vi "USB Config low.vi"(0 "Port":refnum<visa-resource-name>, 1 "Tx msg cluster":T1={"dest"=1, "A/D/C/I"="A", "R/W"="R", "chan"=1, "val (float)"=0.0}, 2 "Error in":errorcluster) -> (3 "Port out":refnum<visa-resource-name>, 4 "Value returned":sgl, 6 "Error out":errorcluster)   [LabVIEW 2018]
uses:
  ctls/muCTA_USB Tx msg cluster.ctl
panel:
  out "Bytes returned":u32
  out "Read buffer (hex)":string
  out "Write buffer (hex)":string
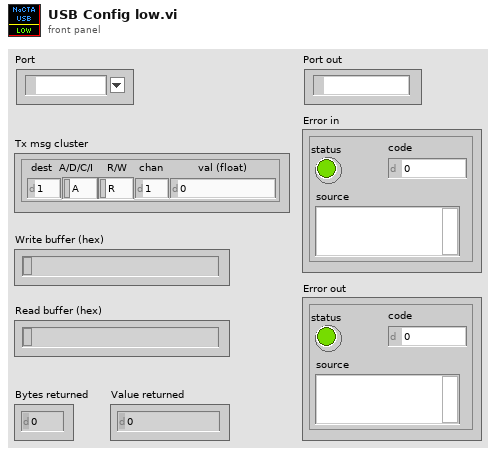
[diagram p1: front panel]
types:
  T1 = typedef "muCTA_USB Tx msg cluster.ctl" = cluster{"dest":u8, "A/D/C/I":string, "R/W":string, "chan":u8, "val (float)":sgl}
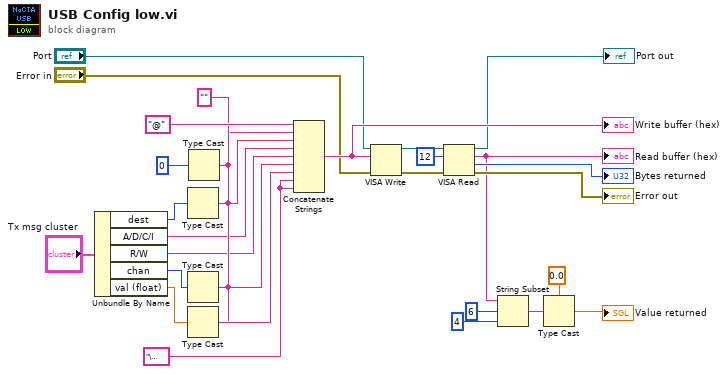
[diagram p0: block diagram]
diagram:
  w24 = "\u0000"
  w18 = ""
  n1 = Unbundle By Name("Tx msg cluster") -> ("dest"=w15:u8, "A/D/C/I"=w14:string, "R/W"=w13:string, "chan"=w12:u8, "val (float)"=w11:sgl)
  n2 = Type Cast(type=w18, x=w15) -> (*(type *) &x=w27:string)
  n3 = Type Cast(type=w18, x=w12) -> (*(type *) &x=w26:string)
  n4 = Type Cast(type=w18, x=w11) -> (*(type *) &x=w25:string)
  n5 = Type Cast(type=w18, x=u8 0) -> (*(type *) &x=w17:string)
  n6 = Concatenate Strings("@", w17, w27, w14, w13, w26, w25, w24, w24) -> (w23:string)
  "Write buffer (hex)" <- w23
  n7 = VISA Write(VISA resource name="Port", write buffer=w23, error in (no error)="Error in") -> (VISA resource name out=w19:refnum<visa-resource-name>, error out=w22:errorcluster)  [unwired: 1 out]
  n8 = VISA Read(VISA resource name=w19, byte count=u32 12, error in (no error)=w22) -> (VISA resource name out=→"Port out":refnum<visa-resource-name>, read buffer=w3:string, return count=→"Bytes returned":u32, error out=→"Error out":errorcluster)
  "Read buffer (hex)" <- w3
  n9 = String Subset(string=w3, offset (0)=6, length (rest)=4 ("length (rest)")) -> (substring=w8:string)
  n10 = Type Cast(type=sgl 0.0, x=w8) -> (*(type *) &x=→"Value returned":sgl)
